vi "Robot Main.vi"() -> ()   [LabVIEW 2012]
doc: "This VI imlements the framework and scheduler for your robotics program. It should not be necessary to modify the framework. You are expected to add your code to the VIs called from Robot Main, the ones located in the Team Code within the project."
uses:
  <vilib>/Rock Robotics/WPI/Camera/WPI_CameraImageSize.ctl
  All_Commands.ctl
  Cirular Shooter/circular_shooter_commands.ctl
  Climber/Climber_Commands.ctl
  All_Outputs.ctl
  Cirular Shooter/Shooter_Outputs.ctl
  Climber/Climber_Outputs.ctl
  All_Sensor_Readings.ctl
  Climber/climber_sensor_readings.ctl
  Cirular Shooter/Shooter_inputs.ctl
  Field Drive/Field_Drive_out.ctl
  <vilib>/Platform/TimedLoop/XDataNode/timing_clust.ctl
  <vilib>/Platform/TimedLoop/XDataNode/nitl_modes.ctl
  <vilib>/Platform/TimedLoop/XDataNode/wakeup.ctl
  Robot Global Data.vi
  <vilib>/Platform/TimedLoop/XDataNode/XDataNode.xnode
  <vilib>/Platform/TimedLoop/XDataNode/XDNodeRunTimeDep.lvlib
panel:
  out "All_Sensor_Readings":T1
  out "All_Outputs":T5
  out "All Driver Commands":T8
  in  "Image Size":T11=enum."320x240"
  in  "Enable Vision":bool
  in  "Finish":bool
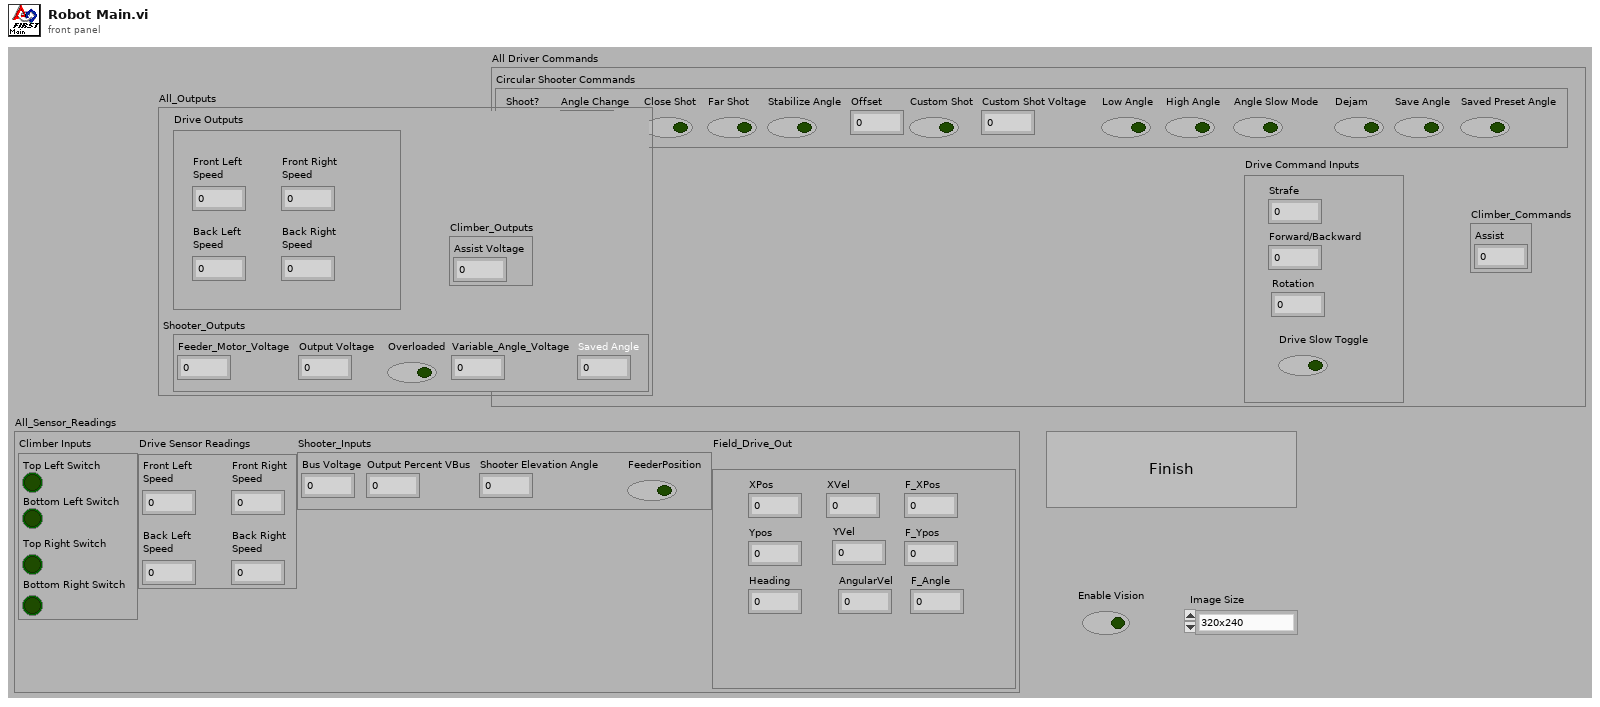
[diagram p1: front panel]
types:
  T1 = typedef "All_Sensor_Readings.ctl" = cluster{"Climber Inputs":T2, "Drive Sensor Readings":cluster{"Front Left\nSpeed":dbl, "Back Left\nSpeed":dbl, "Front Right\nSpeed":dbl, "Back Right\nSpeed":dbl}, "Shooter_Inputs":T3, "Field_Drive_Out\n":T4}
  T2 = typedef "climber_sensor_readings.ctl" = cluster{"Top Left Switch":bool, "Bottom Left Switch":bool, "Top Right Switch":bool, "Bottom Right Switch":bool}
  T3 = typedef "Shooter_inputs.ctl" = cluster{"Bus Voltage":dbl, "Output Percent VBus":dbl, "Shooter Elevation Angle":dbl, "FeederPosition":bool}
  T4 = typedef "Field_Drive_out.ctl" = cluster{"XPos":dbl, "Ypos":dbl, "XVel":dbl, "YVel":dbl, "Heading":dbl, "AngularVel":dbl, "F_XPos":dbl, "F_Ypos":dbl, "F_Angle":dbl}
  T5 = typedef "All_Outputs.ctl" = cluster{"Drive Outputs":cluster{"Front Left\nSpeed":dbl, "Back Left\nSpeed":dbl, "Front Right\nSpeed":dbl, "Back Right\nSpeed":dbl}, "Shooter_Outputs":T6, "Climber_Outputs":T7}
  T6 = typedef "Shooter_Outputs.ctl" = cluster{"Feeder_Motor_Voltage":dbl, "Output Voltage":dbl, "Overloaded":bool, "Variable_Angle_Voltage":dbl, "Saved Angle":dbl}
  T7 = typedef "Climber_Outputs.ctl" = cluster{"Assist Voltage":dbl}
  T8 = typedef "All_Commands.ctl" = cluster{"Circular Shooter Commands":T9, "Drive Command Inputs":cluster{"Strafe":dbl, "Forward/Backward":dbl, "Rotation":dbl, "Drive Slow Toggle":bool}, "Climber_Commands":T10}
  T9 = typedef "circular_shooter_commands.ctl" = cluster{"Shoot?":bool, "Angle Change":dbl, "Close Shot":bool, "Far Shot":bool, "Stabilize Angle ":bool, "Offset":dbl, "Custom Shot":bool, "Custom Shot Voltage":dbl, "Low Angle":bool, "High Angle":bool, "Angle Slow Mode":bool, "Dejam":bool, "Save Angle":bool, "Saved Preset Angle":bool}
  T10 = typedef "Climber_Commands.ctl" = cluster{"Assist":dbl}
  T11 = typedef "WPI_CameraImageSize.ctl" = enum16{"640x480", "320x240", "160x120"}
  T12 = typedef "XDNodeRunTimeDep.lvlib/timing_clust.ctl" = cluster{"Expected End [f-1]":u64, "Actual End [f-1]":u64, "Finished Late? [f-1]":bool, "Expected End [i-1]":u64, "Actual End [i-1]":u64, "Finished Late? [i-1]":bool, "Expected Start [i]":u64, "Actual Start [i]":u64, "Expected Start [f]":u64, "Actual Start [f]":u64, "Source Name":string, "Structure Name":string, "Period":i64, "Deadline":i64, "Offset":i64, "Start":i64, "Priority":i32, "Timeout":i32, "Mode":T13, "Wakeup Reason":T14, "Error":errorcluster, "Source Type":string, "Secondary Source Type":string, "Global End Time":u64, "Global Start Time":u64, "Frame Duration":u64, "Iteration Duration":u64, "Assigned CPU":i32, "I/O Scan Engine Mode":u32}
  T13 = typedef "XDNodeRunTimeDep.lvlib/nitl_modes.ctl" = enum32{"No Change", "Process missed periods, maintain original phase", "Discard missed periods, maintain original phase", "Process missed periods, ignore original phase", "Discard missed periods, ignore original phase"}
  T14 = typedef "XDNodeRunTimeDep.lvlib/wakeup.ctl" = enum32{"Normal", "Aborted", "Asynchronous wakeup", "Timing source error", "Timed loop error", "Timeout"}
  T15 = typedef "Joystick_Inputs.ctl" = cluster{"Joystick 1":cluster{"Axes":cluster{"axis 1 (x)":dbl, "axis 2 (y)":dbl, "axis 3 (throttle)":dbl, "axis 4":dbl, "axis 5":dbl, "axis 6":dbl}, "Buttons":T16}, "Joystick 2":cluster{"Axes":cluster{"axis 1 (x)":dbl, "axis 2 (y)":dbl, "axis 3 (throttle)":dbl, "axis 4":dbl, "axis 5":dbl, "axis 6":dbl}, "Buttons":T16}, "Joystick 3":cluster{"Axes":cluster{"axis 1 (x)":dbl, "axis 2 (y)":dbl, "axis 3 (throttle)":dbl, "axis 4":dbl, "axis 5":dbl, "axis 6":dbl}, "Buttons":T16}, "Joystick 4":cluster{"Axes":cluster{"axis 1 (x)":dbl, "axis 2 (y)":dbl, "axis 3 (throttle)":dbl, "axis 4":dbl, "axis 5":dbl, "axis 6":dbl}, "Buttons":T16}}
  T16 = typedef "WPI_JoystickButtonState.ctl" = cluster{"Button 1":bool, "Button 2":bool, "Button 3":bool, "Button 4":bool, "Button 5":bool, "Button 6":bool, "Button 7":bool, "Button 8":bool, "Button 9":bool, "Button 10":bool, "Button 11":bool, "Button 12":bool}
  T17 = typedef "WPI_DriverStationMatch Info.ctl" = cluster{"Autonomous Elapsed Seconds":dbl, "TeleOp Elapsed Seconds":dbl, "Disabled Elapsed Seconds":dbl, "Visited Autonomous":bool, "Visited TeleOp":bool, "Visited Disabled":bool, "Autonomous Settings":cluster{"Autonomous Style":enum16{"Iterative", "Independent"}, "VI Refnum":refnum<vi>}}
  T18 = typedef "WPI_DriverStationDerivedRobotMode.ctl" = enum16{"Init", "Execute", "Stop"}
  T19 = typedef "WPI_DriverStationRobotMode.ctl" = enum16{"Autonomous Disabled", "Autonomous Enabled", "Teleop Disabled", "Teleop Enabled", "Timeout", "Finish"}
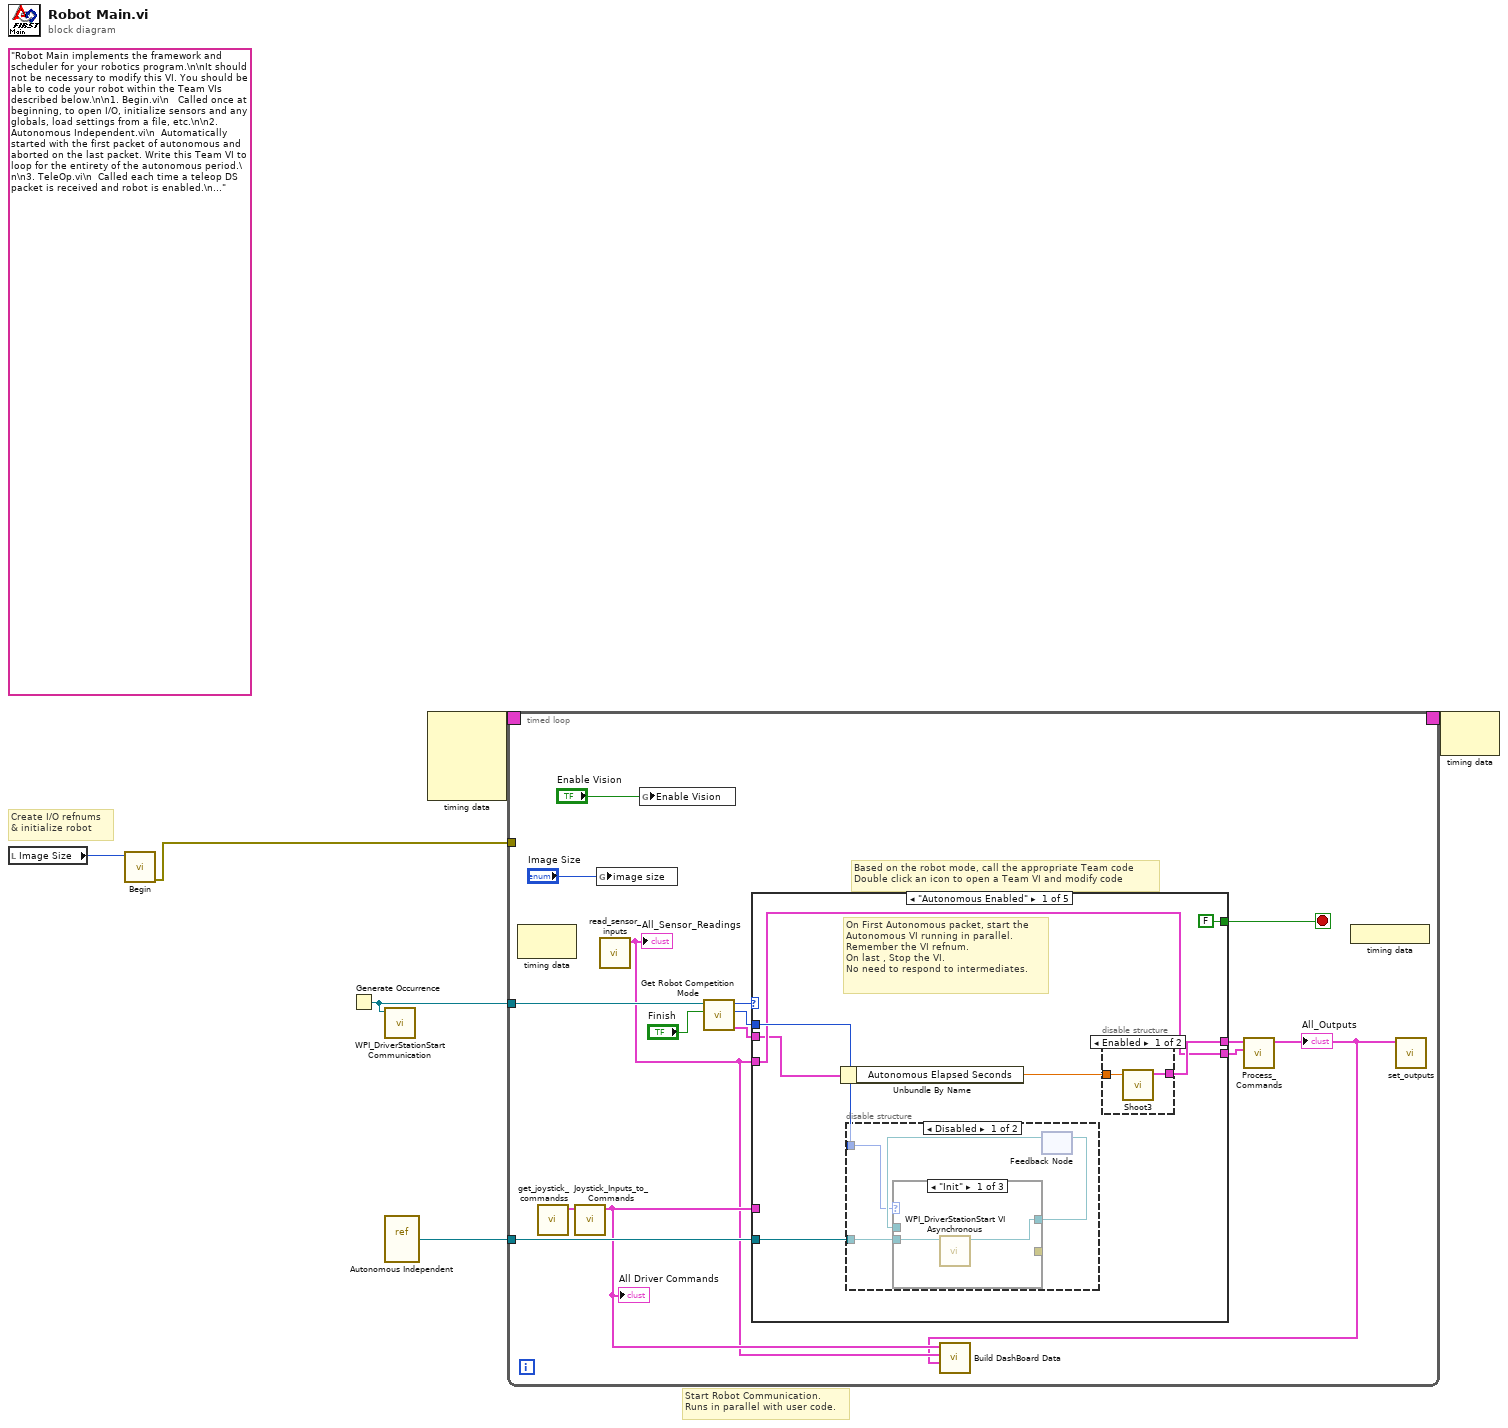
[diagram p0: block diagram]
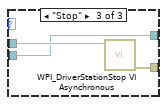
[diagram p3: hidden frame]
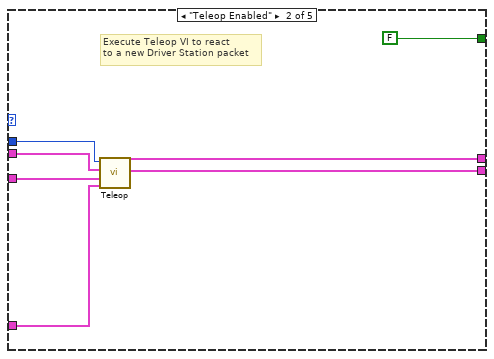
[diagram p6: hidden frame]
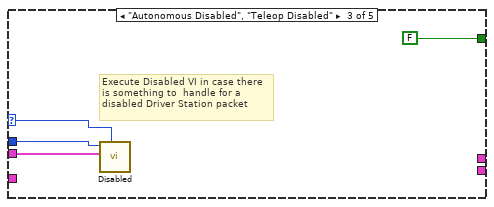
[diagram p7: hidden frame]
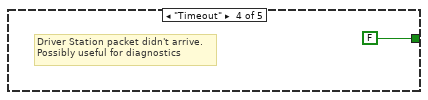
[diagram p8: hidden frame]
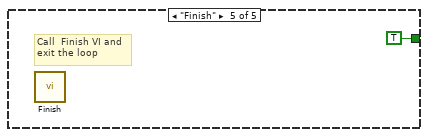
[diagram p9: hidden frame]
diagram:
  (unwired) "Robot Main implements the framework and scheduler for your robotics program.\n\nIt should not be necessary to modify this VI. You should be able to code your robot within the Team VIs described below.\n\n1. Begin.vi\n   Called once at beginning, to open I/O, initialize sensors and any globals, load settings from a file, etc.\n\n2. Autonomous Independent.vi\n  Automatically started with the first packet of autonomous and aborted on the last packet. Write this Team VI to loop for the entirety of the autonomous period.\n\n3. TeleOp.vi\n  Called each time a teleop DS packet is received and robot is enabled.\n\n4. Disabled.vi\n  Called each time a packet is received and the robot is disabled.\n\n5. Vision.vi\n  A parallel loop that acquires and processes camera images.\n\n6. PeriodicTasks.vi\n  Parallel loops running at user-defined rates.\n\n7. Finish.vi\n  Called before exiting, so you can save data, clean up I/O, etc.\n\n8. Build DashBoard Data.vi\n  Called for each driver station packet including timeouts. It is used to send select I/O values back to the Dashboard."
  # "Create I/O refnums\n& initialize robot"
  # "Start Robot Communication.\nRuns in parallel with user code."
  n1 = local read "Image Size"() -> (w5:T11)
  n2 = call "Begin.vi"("Image Size"=w5) -> ("error out"=w1:errorcluster)  [unwired: 10 out]
  n3 = Generate Occurrence() -> (w6:refnum<k4>)
  n4 = call <vilib>:"WPI_DriverStationStart Communication.vi"("occurrence"=w6) -> ()  [unwired: 11 out]
  n5 = vi-ref "Autonomous Independent.vi"() -> (w4:refnum<vi>)
  n6 = node-c288() -> (w3:T12)  [unwired: 4 in]
  n7 = timed-loop {
    tunnel: w6 -> [w19]
    tunnel: w4 -> [w14]
    timing: w3 -> [_]
    timing-out: [_] -> w2
    tunnel: w1 -> [_]
    stop <- w16 stop-if-true
    # "Based on the robot mode, call the appropriate Team code\nDouble click an icon to open a Team VI and modify code"
    n8 = node-c288() -> ()  [unwired: 1 in, 1 out]
    n9 = call "get_joystick_commandss.vi"() -> ("Driver Inputs"=w12:T15)  [unwired: 11 in]
    n10 = call "Joystick_Inputs_to_Commands.vi"("Joystick Inputs"=w12) -> ("All Commands"=w9:T8)  [unwired: 10 in]
    "All Driver Commands" <- w9
    n11 = global write "Robot Global Data.vi" "image size"("Image Size") -> ()
    n12 = call "read_sensor_inputs.vi"() -> ("All_Sensor_Readings"=w8:T1)  [unwired: 11 in]
    "All_Sensor_Readings" <- w8
    n13 = global write "Robot Global Data.vi" "Enable Vision"("Enable Vision") -> ()
    n14 = call "Get Robot Competition Mode.vi"("Finish"="Finish", "DS Occurrence"=w19) -> ("Match Info out"=w17:T17, "Call Context"=w21:T18, "Robot Mode"=w20:T19)  [unwired: 7 out]
    n15 = case shown="\"Autonomous Enabled\"" w20 {
      selector: w20 -> [_ _ w51 _ _]
      tunnel: w21 -> [w29 w49 w53 _ _]
      tunnel: w17 -> [w25 w48 w52 _ _]
      tunnel: [FALSE FALSE FALSE FALSE TRUE] -> w16
      tunnel: w14 -> [w30 _ _ _ _]
      tunnel: w9 -> [_ w45 _ _ _]
      tunnel: [w27 w47 _ _ _] -> w11
      tunnel: w8 -> [w26 w46 _ _ _]
      tunnel: [w26 w43 _ _ _] -> w10
      frame "Autonomous Enabled" {
        # "On First Autonomous packet, start the\nAutonomous VI running in parallel.\nRemember the VI refnum.\nOn last , Stop the VI.\nNo need to respond to intermediates."
        n16 = Unbundle By Name(w25) -> ("Autonomous Elapsed Seconds"=w24:dbl)
        n17 = disable-structure shown="Disabled" {
          disable-tunnel: w30 -> [w32 _]
          disable-tunnel: w29 -> [w31 _]
          frame Disabled {
            n18 = feedback #1() -> (w33:refnum<vi>)  [unwired: 1 out]
            n19 = case shown="\"Init\"" w31 {
              tunnel: w32 -> [w36 _ w39]
              tunnel: [w35 w37 w39] -> w34
              tunnel: w33 -> [_ w37 w40]
              tunnel: [_ _ w38] -> _
              frame "Init" {
                n20 = call <vilib>:"WPI_DriverStationStart VI Asynchronous.vi"("VI"=w36) -> ("VI out"=w35:refnum<vi>)  [unwired: 10 out]
              }
              frame "Execute", Default {
                # "Nothing to do"
              }
              frame "Stop" {
                n21 = call <vilib>:"WPI_DriverStationStop VI Asynchronous.vi"("VI Refnum"=w40) -> ("error out"=w38:errorcluster)  [unwired: 10 out]
              }
            }
            n22 = feedback-in #1(w34) -> ()
          }
          frame Enabled {
          }
        }
        n23 = disable-structure shown="Enabled" {
          disable-tunnel: [w42 _] -> w27
          disable-tunnel: w24 -> [w41 _]
          frame Enabled {
            n24 = call "Shoot3.vi"("Elapsed"=w41) -> ("All Driver Commands"=w42:T8)  [unwired: 10 in]
          }
          frame Disabled {
          }
        }
      }
      frame "Teleop Enabled" {
        # "Execute Teleop VI to react\nto a new Driver Station packet"
        n25 = call "Teleop.vi"("All Driver Commands In"=w45, "All_Sensor_Readings"=w46, "Match Info"=w48, "Call Context"=w49) -> ("All_Sensor_Readings Out"=w43:T1, "All Driver Commands Out"=w47:T8)  [unwired: 6 out]
      }
      frame "Autonomous Disabled", "Teleop Disabled" {
        # "Execute Disabled VI in case there\nis something to  handle for a\ndisabled Driver Station packet"
        n26 = call "Disabled.vi"("Robot Mode"=w51, "Match Info"=w52, "Call Context"=w53) -> ()  [unwired: 1 in, 8 out]
      }
      frame "Timeout" {
        # "Driver Station packet didn't arrive.\nPossibly useful for diagnostics"
      }
      frame "Finish" {
        # "Call  Finish VI and\nexit the loop"
        n27 = call "Finish.vi"() -> ()  [unwired: 1 in, 7 out]
      }
    }
    n28 = call "Process_Commands.vi"("All_Sensor_Readings"=w10, "All Driver Commands"=w11) -> ("All_Outputs"=w7:T5)  [unwired: 9 in]
    "All_Outputs" <- w7
    n29 = call "Build DashBoard Data.vi"("All_Outputs"=w7, "All_Sensor_Readings"=w8, "All Driver Commands"=w9) -> ()  [unwired: 9 out]
    n30 = node-c288() -> ()  [unwired: 1 out]
    n31 = call "set_outputs.vi"("All_Outputs"=w7) -> ()  [unwired: 11 in]
  }
  n32 = node-c288(w2) -> ()  [unwired: 1 out]
